vi "CAN_ReadFrame_Stream.vi"(8 "error in (no error)":errorcluster, 11 "XNET Session":refnum<k21>) -> (0 "error out":errorcluster)   [LabVIEW 2021]
uses:
  <vilib>/xnet/xnet.llb/XNET Frame CAN.ctl
  <vilib>/xnet/xnet.llb/XNET Frame Type CAN.ctl
  <vilib>/xnet/xnet.llb/XNET Read (Frame CAN).vi
  <vilib>/xnet/xnet.llb/XNET Create Session (Conversion).vi
  <vilib>/xnet/xnet.llb/XNET Convert (Frame CAN to Signal).vi
panel:
  out "data":T1[](array[typedef]) {"payload" format="%x"; "timestamp" format="%<%.7X\n%x>T"; "type" items=["CAN Data"=0, "CAN Remote"=1, "CAN Bus Error"=2, "CAN 2.0 Data"=8, "CAN FD Data"=16, "CAN FD+BRS Data"=24, "J1939 Data"=192, "Delay"=224, "Log Trigger"=225, "Start Trigger"=226]; "identifier" format="%x"}
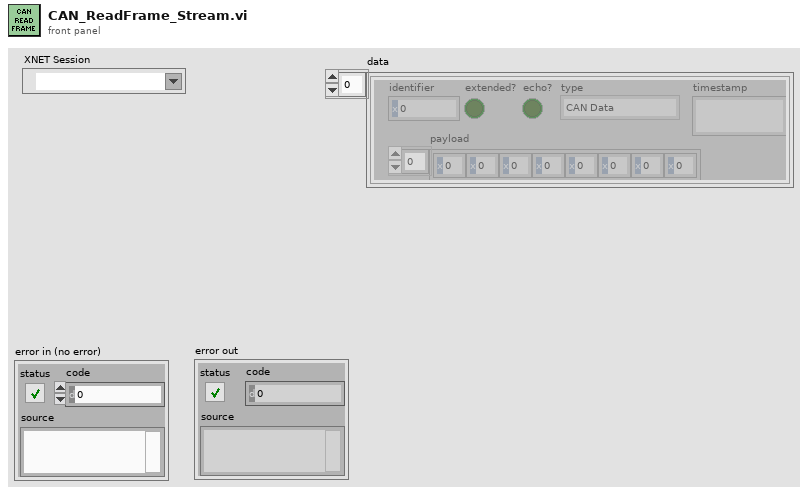
[diagram p1: front panel]
types:
  T1 = typedef "XNET Frame CAN.ctl" = cluster{"timestamp":timestamp, "payload":u8[], "identifier":u32, "type":T2, "extended?":bool, "echo?":bool}
  T2 = typedef "XNET Frame Type CAN.ctl" = u8
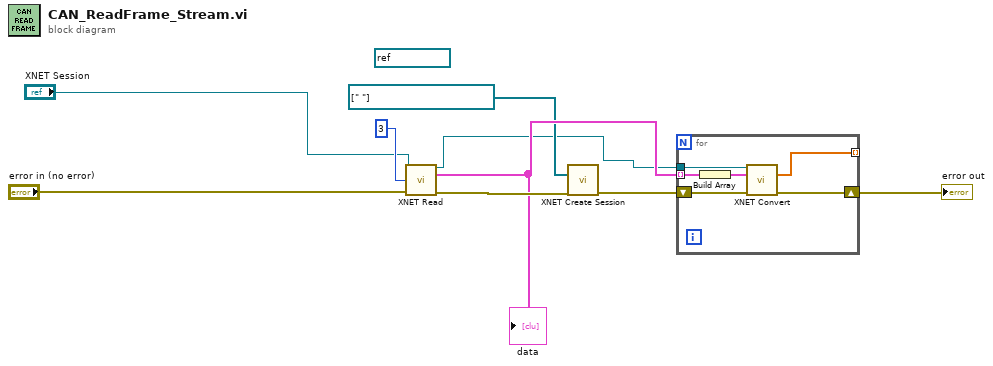
[diagram p0: block diagram]
diagram:
  (unwired) refnum<k21> "Database" ("XNET Database")
  n1 = call-poly <vilib>:"XNET Read.vi"("session in"="XNET Session", "number to read (-1)"=3, "error in (no error)"="error in (no error)") -> ("session out"=w1:refnum<k21>, "data"=w5:T1[], "error out"=w6:errorcluster)  [unwired: 9 in, 1 out]
  "data" <- w5
  n2 = call-poly <vilib>:"XNET Create Session.vi"("signal list"=refnum<k21>[] [" "], "error in (no error)"=w6) -> ("error out"=w9:errorcluster)  [unwired: 12 in, 1 out]
  n3 = for {
    tunnel: w1 -> [w14]
    tunnel: w5 -> [w12] mode=indexing
    shift-right: [w13] -> w7
    shift-left: w9 -> [w15]
    tunnel: [w10] -> _ mode=indexing
    n4 = Build Array(w12) -> (w11:T1[])
    n5 = call-poly <vilib>:"XNET Convert.vi"("session in"=w14, "frame data"=w11, "error in (no error)"=w15) -> ("signal data"=w10:dbl[], "error out"=w13:errorcluster)  [unwired: 10 in, 1 out]
  }
  "error out" <- w7
